vi "NavDisplay Init.vi"(10 "Application Directory":path) -> (2 "roll image":T1, 3 "pitch image":T1)   [LabVIEW 8.6]
uses:
  <vilib>/picture/picture.llb/imagedata.ctl
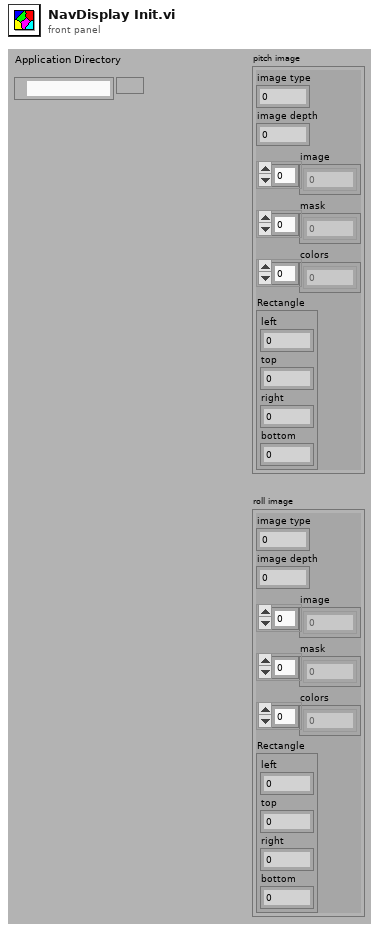
[diagram p1: front panel]
types:
  T1 = typedef "imagedata.ctl" = cluster{"image type":i32, "image depth":i32, "image":u8[], "mask":u8[], "colors":u32[], "Rectangle":cluster{"left":i16, "top":i16, "right":i16, "bottom":i16}}
  T2 = cluster{"left":i16, "top":i16, "right":i16, "bottom":i16}
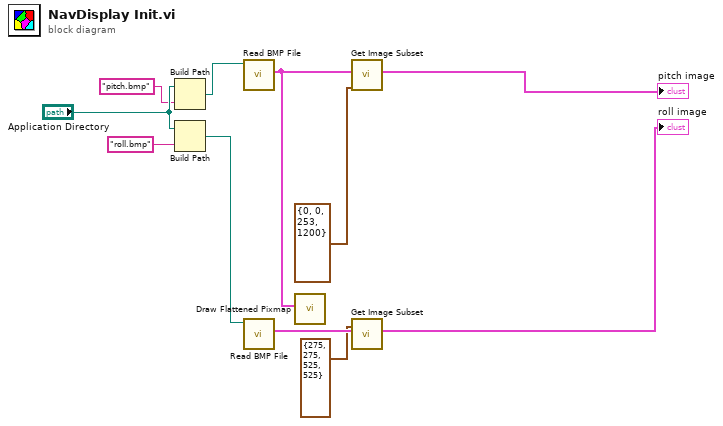
[diagram p0: block diagram]
diagram:
  n1 = Build Path(base path="Application Directory", name or relative path="pitch.bmp") -> (appended path=w2:path)
  n2 = Build Path(base path="Application Directory", name or relative path="roll.bmp") -> (appended path=w7:path)
  n3 = call <vilib>:"Read BMP File.vi"("path to BMP file"=w2) -> ("image data"=w4:T1)  [unwired: 1 in, 9 out]
  n4 = call <vilib>:"Read BMP File.vi"("path to BMP file"=w7) -> ("image data"=w8:T1)  [unwired: 1 in, 9 out]
  n5 = call <vilib>:"Draw Flattened Pixmap.vi"("image data"=w4) -> ()  [unwired: 1 in, 8 out]
  n6 = call <vilib>:"Get Image Subset.vi"("subset rect"=T2 {"left"=0, "top"=0, "right"=253, "bottom"=1200}, "image data"=w4) -> ("image subset"=→"pitch image":T1)  [unwired: 5 out]
  n7 = call <vilib>:"Get Image Subset.vi"("subset rect"=T2 {"left"=275, "top"=275, "right"=525, "bottom"=525}, "image data"=w8) -> ("image subset"=→"roll image":T1)  [unwired: 5 out]
